vi "上位机.vi"() -> ()   [LabVIEW 2016]
doc: "This example demonstrates the Traditional MeanShift algorithm to track an object in the image."
uses:
  <vilib>/vision/driver/NI_Vision_Acquisition_Software.lvlib
  <vilib>/userdefined/High Color/IMAQdx.ctl
panel:
  in  "选择区域标志位":bool
  in  "是否删除跟踪对象？":bool
  out "运动目标跟踪云台系统":T1(plugin-control)
  in  "Stop":bool
  in  "Delay (s.)":dbl(slide) scale=0.0..2.0
  # "Overview: Demonstrate the Traditional MeanShift algorithm to track an object in the image.\nRequirements: LabVIEW Full Development System and Vision Development Module.\nInstructions: Run the VI."
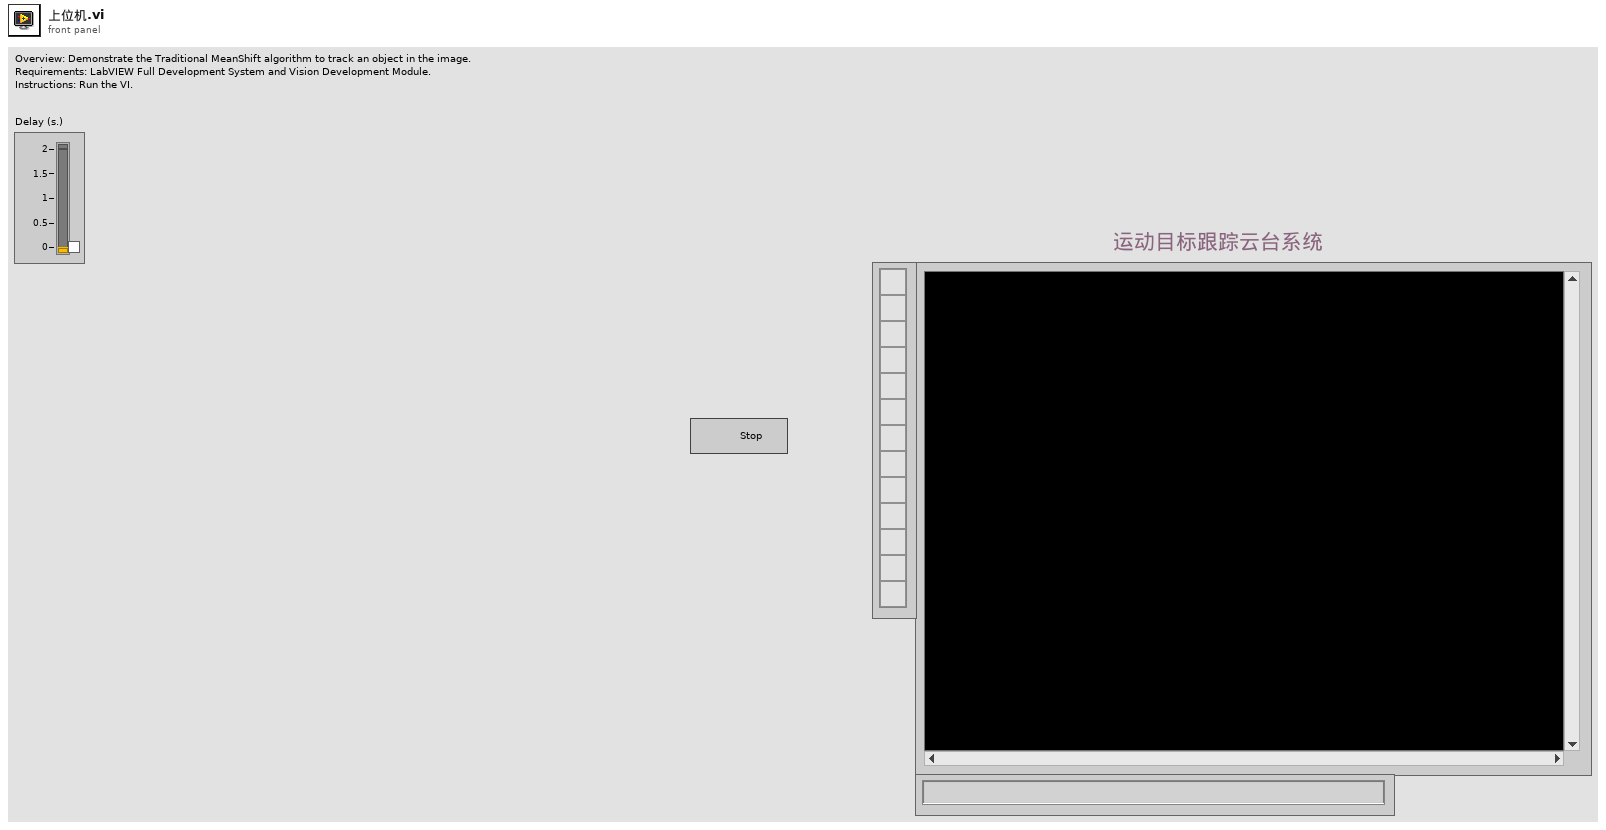
[diagram p1: front panel]
types:
  T1 = typedef "IMAQ Image.ctl" = refnum<image>
  T2 = typedef "IMAQdx.ctl" = refnum<k21>
  T3 = cluster{"Number of Histogram Bins":i32, "Blending Parameter (%)":dbl, "Maximum Iterations":i32}
  T4 = typedef "Image Type" = u32
  T5 = typedef "IMAQ Object Tracking Session.ctl" = refnum<k20>
  T6 = cluster{"Global Rectangle":i32[], "Contours":cluster{"Contour Type":u32, "ROI Type":u32, "Points":i32[]}[]}
  T7 = cluster{"Label":string, "Score":i32, "Angle":dbl, "Location":cluster{"X":dbl, "Y":dbl}, "Bounding Box":cluster{"X":dbl, "Y":dbl}[], "Object Found?":bool}[]
  T8 = cluster{"Label":string, "Score":i32, "Angle":dbl, "Location":cluster{"X":dbl, "Y":dbl}, "Bounding Box":cluster{"X":dbl, "Y":dbl}[], "Object Found?":bool}
  T9 = typedef "ROI Descriptor" = cluster{"Global Rectangle":i32[], "Contours":cluster{"ID":enum32{"External", "Internal"}, "Type":u32, "Coordinates":i32[]}[]}
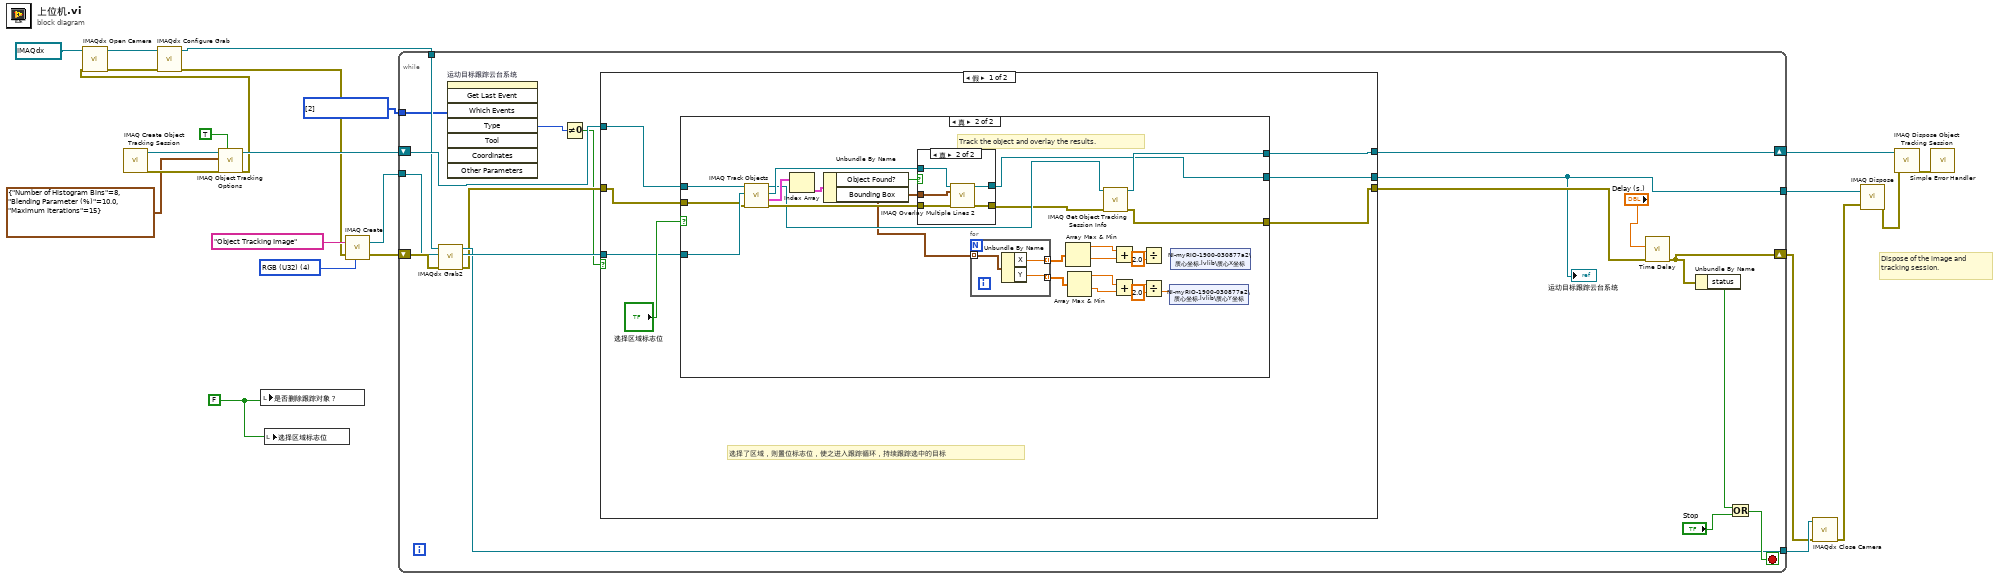
[diagram p0: block diagram]
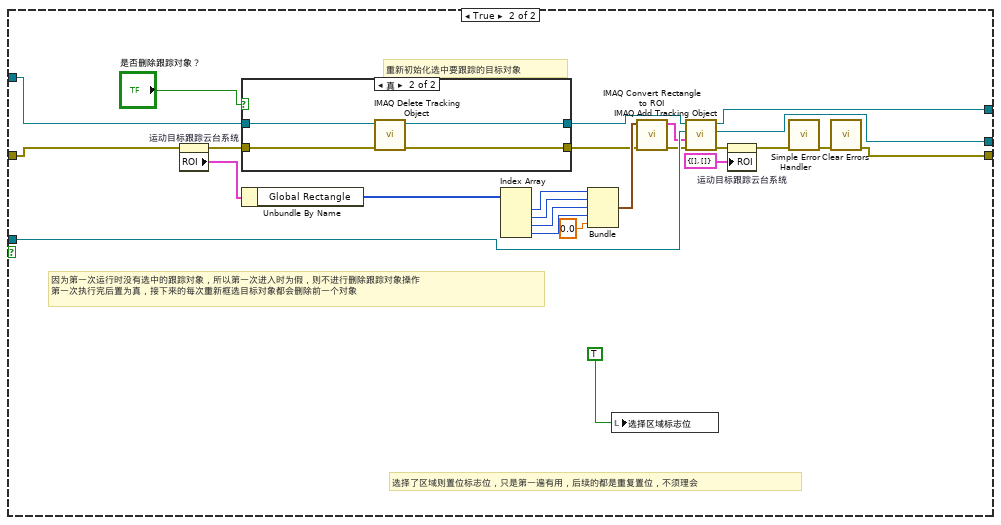
[diagram p4: hidden frame]
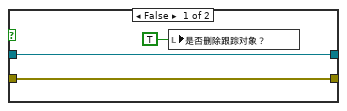
[diagram p5: hidden frame]
diagram:
  w1 = FALSE ("空白按钮")
  w3 = i32[] [2] items=["No Event"=0, "Click Event"=1, "Draw Event"=2, "Size Event"=4, "Scroll Event"=5, "Double Click Event"=8] ("Which Events")
  w15 = T4 4 items=["Grayscale (U8)", "Grayscale (I16)", "Grayscale (SGL)", "Complex (CSG)", "RGB (U32)", "HSL (U32)", "RGB (U64)", "Grayscale (U16)"] ("Image Type")
  # "Dispose of the image and tracking session."
  n1 = call "IMAQ Create Object Tracking Session"() -> ("error out"=w17:errorcluster, "Object Tracking Session"=w20:T5)  [unwired: 1 in, 9 out]
  n2 = call-poly "IMAQ Object Tracking Options"("Get/Set (Get)"=TRUE, "error in (no error)"=w17, "Mean Shift Options in"=T3 {"Number of Histogram Bins"=8, "Blending Parameter (%)"=10.0, "Maximum Iterations"=15}, "Object Tracking Session In"=w20) -> ("error out"=w9:errorcluster, "Object Tracking Session Out"=w19:T5)  [unwired: 5 in, 1 out]
  n3 = call <vilib>:"IMAQdx Open Camera.vi"("error in"=w9, "Session In"=T2 "cam1") -> ("error out"=w10:errorcluster, "Session Out"=w11:T2)  [unwired: 8 in]
  n4 = call <vilib>:"IMAQdx Configure Grab.vi"("error in"=w10, "Session In"=w11) -> ("error out"=w8:errorcluster, "Session Out"=w7:T2)  [unwired: 8 in]
  n5 = local write "是否删除跟踪对象？"(w1) -> ()
  n6 = local write "选择区域标志位"(w1) -> ()
  n7 = call "IMAQ Create"("Image Name"="Object Tracking Image", "Image Type"=w15, "error in (no error)"=w8) -> ("New Image"=w14:T1, "error out"=w13:errorcluster)  [unwired: 2 in]
  n8 = while {
    tunnel: [w26] -> w24
    shift-right: [w40] -> w23
    shift-left: w19 -> [w41]
    tunnel: w14 -> [w32]
    shift-right: [w36] -> w5
    shift-left: w13 -> [w33]
    tunnel: [w30] -> w6
    tunnel: w7 -> [w34]
    tunnel: w3 -> [w28]
    stop <- w35 stop-if-true
    n9 = call <vilib>:"IMAQdx Grab2.vi"("error in"=w33, "Image In"=w32, "Session In"=w34) -> ("error out"=w29:errorcluster, "Image Out"=w31:T1, "Session Out"=w30:T2)  [unwired: 5 in, 1 out]
    n10 = invoke on="运动目标跟踪云台系统" class="ImageControl" method="Get Last Event"("Which Events"=w28) -> ("Type"=w27:i32)  [unwired: 7 in, 7 out]
    n11 = Not Equal To 0?(x=w27) -> (x != 0?=w25:bool)
    n12 = case shown="假" w25 {
      tunnel: [w43 w112] -> w26
      tunnel: w41 -> [w48 w111]
      tunnel: [w45 w110] -> w40
      tunnel: [w44 w109] -> w38
      tunnel: w31 -> [w47 w108]
      tunnel: w29 -> [w46 w107]
      frame False {
        # "选择了区域，则置位标志位，使之进入跟踪循环，持续跟踪选中的目标"
        n13 = case shown="真" "选择区域标志位" {
          tunnel: w48 -> [w52 w70]
          tunnel: w47 -> [w51 w69]
          tunnel: w46 -> [w50 w68]
          tunnel: [w52 w67] -> w45
          tunnel: [w50 w66] -> w44
          tunnel: [w51 w65] -> w43
          frame False {
          }
          frame True {
            # "Track the object and overlay the results."
            n14 = call "IMAQ Track Objects"("error in (no error)"=w68, "Image"=w69, "Object Tracking Session In"=w70) -> ("error out"=w75:errorcluster, "Objects (pixel)"=w77:T7, "Image (duplicate)"=w76:T1, "Object Tracking Session Out"=w72:T5)  [unwired: 1 in, 4 out]
            n15 = Index Array(array=w77) -> (element=w74:T8)  [unwired: 1 in]
            n16 = Unbundle By Name(w74) -> ("Object Found?"=w73:bool, "Bounding Box"=w64:cluster{"X":dbl, "Y":dbl}[])
            n17 = case shown="真" w73 {
              tunnel: w76 -> [w81 w87]
              tunnel: [w81 w86] -> w65
              tunnel: w64 -> [_ w85]
              tunnel: w75 -> [w82 w84]
              tunnel: [w82 w83] -> w71
              frame False {
              }
              frame True {
                n18 = call "IMAQ Overlay Multiple Lines 2"("Image"=w87, "Line End Points"=w85, "error in (no error)"=w84) -> ("Image Out"=w86:T1, "error out"=w83:errorcluster)  [unwired: 5 in, 6 out]
              }
            }
            n19 = for {
              tunnel: w64 -> [w80] mode=indexing
              tunnel: [w79] -> w63 mode=indexing
              tunnel: [w78] -> w62 mode=indexing
              n20 = Unbundle By Name(w80) -> ("X"=w79:dbl, "Y"=w78:dbl)
            }
            n21 = Array Max & Min(array=w63) -> (max value=w61:dbl, min value=w60:dbl)  [unwired: 2 out]
            n22 = Array Max & Min(array=w62) -> (max value=w55:dbl, min value=w54:dbl)  [unwired: 2 out]
            n23 = call "IMAQ Get Object Tracking Session Info"("error in (no error)"=w71, "Object Tracking Session In"=w72) -> ("error out"=w66:errorcluster, "Object Tracking Session Out"=w67:T5)  [unwired: 6 in, 2 out]
            n24 = Add(x=w61, y=w60) -> (x+y=w59:dbl)
            n25 = Add(x=w55, y=w54) -> (x+y=w56:dbl)
            n26 = Divide(x=w59, y=2.0) -> ()  [unwired: 1 out]
            n27 = Divide(x=w56, y=2.0) -> (x/y=w53:dbl)
            n28 = shared-variable "NI-myRIO-1900-030877a2\\质心坐标.lvlib\\质心Y坐标"(w53) -> ()  [unwired: 1 in, 1 out]
            n29 = shared-variable "NI-myRIO-1900-030877a2\\质心坐标.lvlib\\质心X坐标"() -> ()  [unwired: 2 in, 1 out]
          }
        }
      }
      frame True {
        # "选择了区域则置位标志位，只是第一遍有用，后续的都是重复置位，不须理会"
        # "因为第一次运行时没有选中的跟踪对象，所以第一次进入时为假，则不进行删除跟踪对象操作\n第一次执行完后置为真，接下来的每次重新框选目标对象都会删除前一个对象"
        # "重新初始化选中要跟踪的目标对象"
        n30 = property on="运动目标跟踪云台系统" class="ImageControl"(error in=w107) -> (error out=w96:errorcluster, "ROI"=w104:T6)  [unwired: 1 in, 1 out]
        n31 = case shown="真" "是否删除跟踪对象？" {
          tunnel: w96 -> [w115 w117]
          tunnel: [w115 w116] -> w95
          tunnel: w111 -> [w114 w118]
          tunnel: [w114 w119] -> w94
          frame False {
            n32 = local write "是否删除跟踪对象？"(TRUE ("空白按钮")) -> ()
          }
          frame True {
            n33 = call "IMAQ Delete Tracking Object"("error in (no error)"=w117, "Object Tracking Session In"=w118) -> ("error out"=w116:errorcluster, "Object Tracking Session Out"=w119:T5)  [unwired: 8 in]
          }
        }
        n34 = Unbundle By Name(w104) -> ("Global Rectangle"=w103:i32[])
        n35 = Index Array(array=w103) -> (element #1=w102:i32, element #2=w101:i32, element #3=w100:i32, element #4=w99:i32)  [unwired: 4 in]
        n36 = Bundle(w102, w101, w100, w99, 0.0) -> (w97:cluster{i32, i32, i32, i32, dbl})  [unwired: 1 in]
        n37 = local write "选择区域标志位"(TRUE ("选择区域标志位")) -> ()
        n38 = call "IMAQ Convert Rectangle to ROI"("error in (no error)"=w95, "Rectangle"=w97) -> ("error out"=w106:errorcluster, "ROI Descriptor"=w105:T9)  [unwired: 7 in]
        n39 = call "IMAQ Add Tracking Object"("error in (no error)"=w106, "ROI Descriptor"=w105, "Image"=w108, "Object Tracking Session In"=w94) -> ("error out"=w93:errorcluster, "Image (duplicate)"=w112:T1, "Object Tracking Session Out"=w110:T5)  [unwired: 1 in, 4 out]
        n40 = property on="运动目标跟踪云台系统" class="ImageControl"(error in=w93, "ROI"=T6 {"Global Rectangle"=[], "Contours"=[]}) -> (error out=w91:errorcluster)  [unwired: 1 in, 1 out]
        n41 = call <vilib>:"Simple Error Handler.vi"("error in (no error)"=w91) -> ("error out"=w90:errorcluster)  [unwired: 4 in, 4 out]
        n42 = call <vilib>:"Clear Errors.vi"("error in (no error)"=w90) -> ("error out"=w109:errorcluster)  [unwired: 5 in, 1 out]
      }
    }
    "运动目标跟踪云台系统" <- w26
    n43 = call "Time Delay"("error in (no error)"=w38, "Delay Time (s)"="Delay (s.)") -> ("error out"=w36:errorcluster)  [unwired: 9 in]
    n44 = Unbundle By Name(w36) -> ("status"=w42:bool)
    n45 = Or(x=w42, y="Stop") -> (x .or. y?=w35:bool)
  }
  n46 = call <vilib>:"IMAQdx Close Camera.vi"("error in"=w5, "Session In"=w6) -> ("error out"=w4:errorcluster)  [unwired: 9 in]
  n47 = call "IMAQ Dispose"("Image"=w24, "error in (no error)"=w4) -> ("error out"=w22:errorcluster)  [unwired: 1 in, 3 out]
  n48 = call "IMAQ Dispose Object Tracking Session"("error in (no error)"=w22, "Object Tracking Session"=w23) -> ("error out"=w21:errorcluster)  [unwired: 9 out]
  n49 = call <vilib>:"Simple Error Handler.vi"("error in (no error)"=w21) -> ()  [unwired: 1 in, 8 out]
